vi "toml_list_files.vi"(8 "error in (no error)":errorcluster) -> (0 "error out":errorcluster, 3 "files loaded":path[](array[path]))   [LabVIEW 2017]
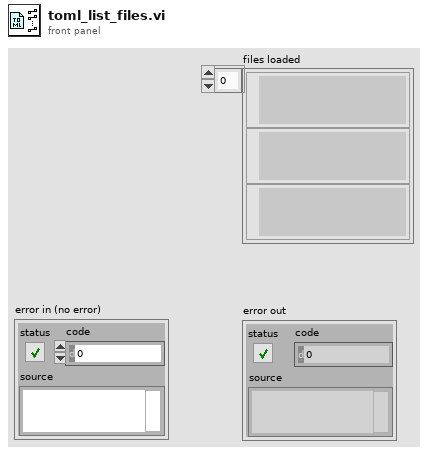
[diagram p1: front panel]
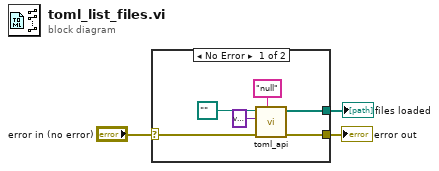
[diagram p0: block diagram]
diagram:
  n1 = case shown="No Error" "error in (no error)" {
    selector: "error in (no error)" -> [w9 w10]
    tunnel: [w5 w10] -> w2
    tunnel: [w4 _] -> w1
    frame No Error {
      n2 = call "toml_api.vi"("cmd"="null", "error in (no error)"=w9, "data in"=variant, "resolved path"=path "" ("path in")) -> ("error out"=w5:errorcluster, "files"=w4:path[])  [unwired: 4 in, 2 out]
    }
    frame Error {
    }
  }
  "error out" <- w2
  "files loaded" <- w1
